vi "Sum array optimised.vi"(1 "Array in":dbl[](array[numeric])) -> (0 "Sum":dbl)   [LabVIEW 2015]
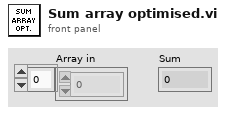
[diagram p1: front panel]
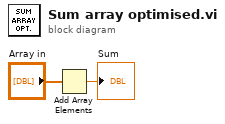
[diagram p0: block diagram]
diagram:
  n1 = Add Array Elements(numeric array="Array in") -> (sum=→"Sum":dbl)
